vi "Vision Processing.vi"(4 "error in (no error)":errorcluster, 5 "Camera Type":enum16{"206", "1011"}(ring)=enum."1011", 6 "Camera Name":string="Camera") -> ()   [LabVIEW 2013]
uses:
  Robot Global Data.vi
  <vilib>/vision/NI_Vision_Development_Module.lvlib
panel:
  out "Target Info":T1(array[cluster])
  in  "Area Size Limit %":dbl=0.5
  in  "Particle Count Limit":i32=8
  in  "Score Limits":T2={"Rect Coverage"=60.0, "X Edge Strength"=40.0, "Y Edge Strength"=60.0, "Center"=75.0, "Outer"=75.0}
  in  "Processing":enum32{"Color", "Monochrome"}(tab)=enum."Monochrome"
  out "Value":cluster{i32, i32}
  out "Saturation":cluster{i32, i32}
  out "Hue":cluster{i32, i32}
  in  "Luminance":i32=255
  in  "Saturation":i32=255
  in  "Hue":i32(knob)=65 scale=0.0..255.0
  in  "Margins":cluster{"Hue":i32, "Sat":i32, "Val":i32}={"Hue"=33, "Sat"=53, "Val"=9} {"Sat" scale=0.0..80.0; "Val" scale=0.0..80.0; "Hue" scale=0.0..80.0}
  in  "Range":cluster{"Lower value":sgl, "Upper value":sgl}={"Lower value"=150.0, "Upper value"=255.0} {"Lower value" scale=0.0..255.0; "Upper value" scale=0.0..255.0}
  in  "View":bool
  out "Processed Image":T3(plugin-control)
  # "Instructions:\nProcessing the reflective tape that is illuminated by a ring light can be based\non color or light intensity.\nParticles within the image are scored by rectangle coverage, aspect ratio, and\nfor being hollow with a bold edge. A particle is considered a target if all scores\nare above the score limits. Particles can be annotated -- surrounded by\na rectangle and scores drawn to the left .\nTo control the number of particles being scored, use the count limit and the size\nlimit."
  # "To debug, Enable using the View button.\nFor color processing, you can click in the image to select the color for processing."
  # "Enable by clicking the View button.\nGreen scores are above the limit, orange are below. Inner/outer rect\nindicates all passed."
  # "Lower/Upper"
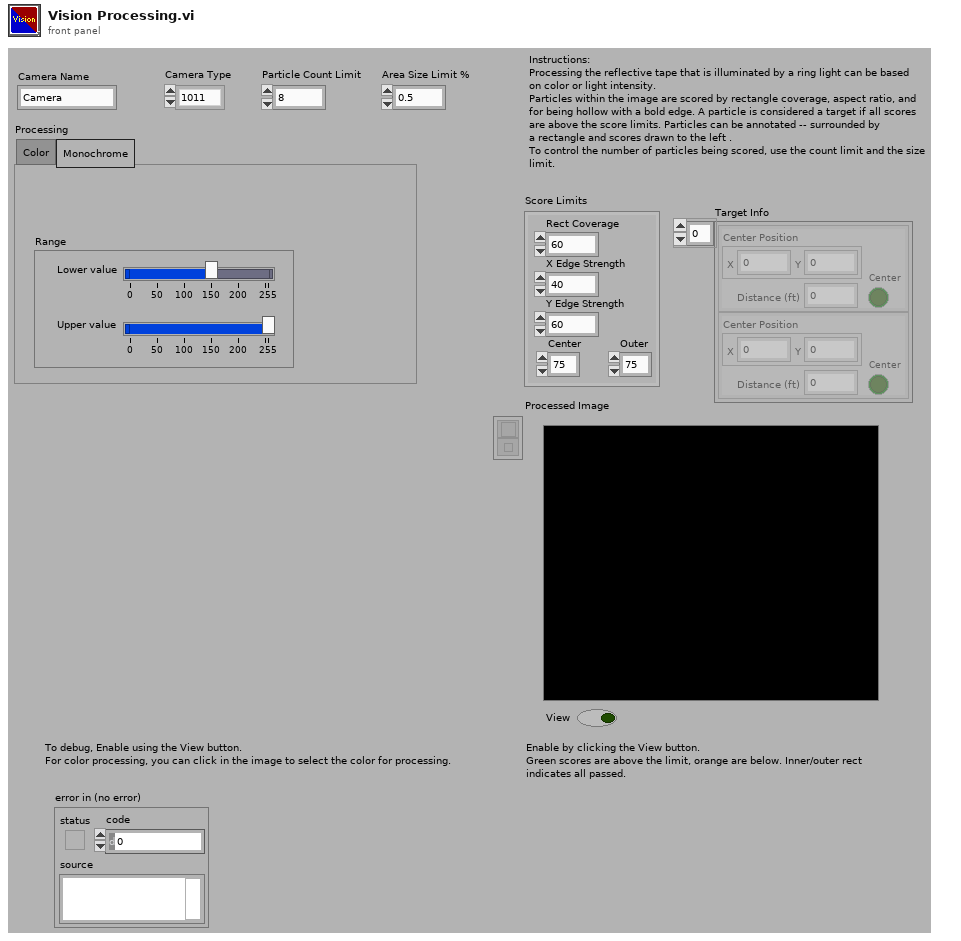
[diagram p1: front panel]
types:
  T1 = cluster{"Center Position":cluster{"X":dbl, "Y":dbl}, "Distance (ft)":dbl, "Center":bool}[]
  T2 = cluster{"Rect Coverage":dbl, "X Edge Strength":dbl, "Y Edge Strength":dbl, "Center":dbl, "Outer":dbl}
  T3 = typedef "IMAQ Image.ctl" = refnum<image>
  T4 = typedef "Image Type" = u32
  T5 = typedef "WPI_CameraDevRef.ctl" = cluster{"Camera Address":string, "CameraStatus":errorcluster, "Acquire Image Notifier":refnum<notifier>}
  T6 = cluster{"Position":cluster{"X":dbl, "Y":dbl}, "Distance (ft)":dbl, "Center":bool}[]
  T7 = typedef "WPI_CameraImageSize.ctl" = enum16{"640x480", "320x240", "160x120"}
  T8 = cluster{cluster{"Left":dbl, "Top":dbl, "Right":dbl, "Bottom":dbl}, "Scores":dbl[], cluster{"Long":dbl, "Short":dbl}}[]
  T9 = cluster{"Target Center (-1 to 1)":cluster{"X":dbl, "Y":dbl}, "Distance (ft)":dbl, "Center Target":bool}
  T10 = cluster{"Target Center (-1 to 1)":cluster{"X":dbl, "Y":dbl}, "Distance (ft)":dbl, "Center Target":bool}[]
  T11 = cluster{"Left":dbl, "Top":dbl, "Right":dbl, "Bottom":dbl}
  T12 = cluster{"Position":cluster{"X":dbl, "Y":dbl}, "Distance (ft)":dbl, "Center":bool}
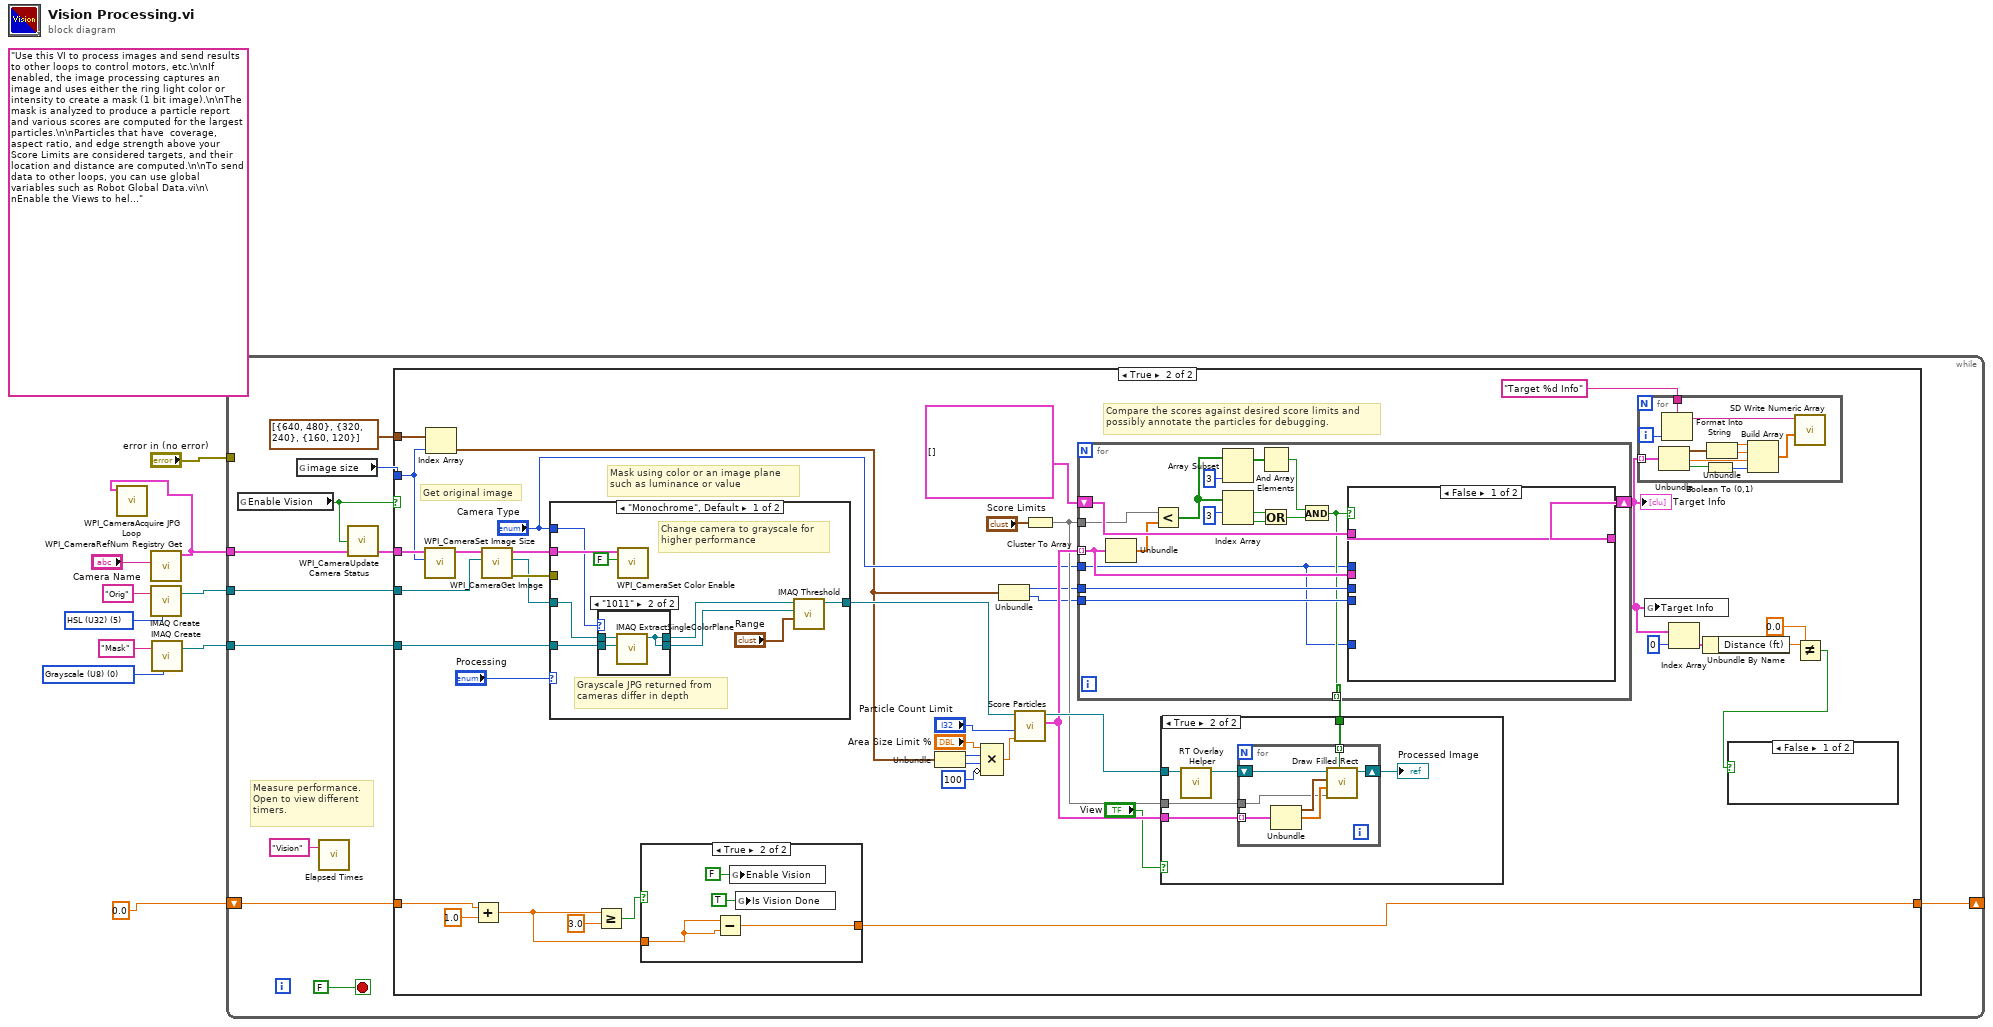
[diagram p0: block diagram]
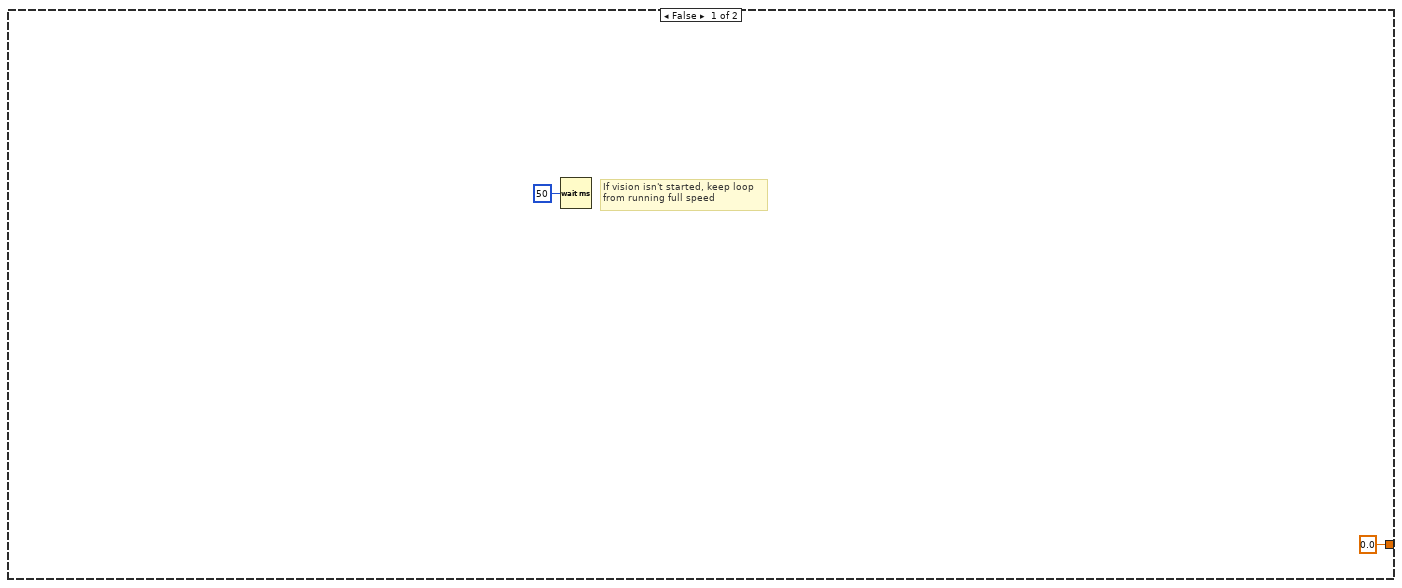
[diagram p2: hidden frame]
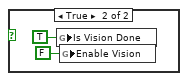
[diagram p3: hidden frame]
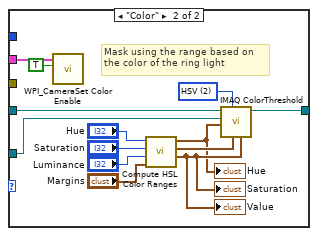
[diagram p6: hidden frame]
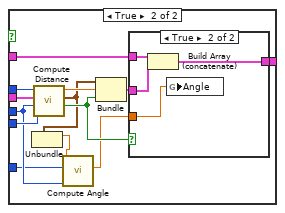
[diagram p8: hidden frame]
diagram:
  w5 = T4 0 items=["Grayscale (U8)", "Grayscale (I16)", "Grayscale (SGL)", "Complex (CSG)", "RGB (U32)", "HSL (U32)", "RGB (U64)", "Grayscale (U16)"] ("Image Type")
  (unwired) "Use this VI to process images and send results to other loops to control motors, etc.\n\nIf enabled, the image processing captures an image and uses either the ring light color or intensity to create a mask (1 bit image).\n\nThe mask is analyzed to produce a particle report and various scores are computed for the largest particles.\n\nParticles that have  coverage, aspect ratio, and edge strength above your Score Limits are considered targets, and their location and distance are computed.\n\nTo send data to other loops, you can use global variables such as Robot Global Data.vi\n\nEnable the Views to help debug color settings. Disable the View to speed up processing."
  w9 = T4 5 items=["Grayscale (U8)", "Grayscale (I16)", "Grayscale (SGL)", "Complex (CSG)", "RGB (U32)", "HSL (U32)", "RGB (U64)", "Grayscale (U16)"] ("Image Type")
  n1 = call <vilib>:"WPI_CameraRefNum Registry Get.vi"("refnum name"="Camera Name") -> ("CameraDevRef"=w1:T5)  [unwired: 9 in, 1 out]
  n2 = call <vilib>:"WPI_CameraAcquire JPG Loop.vi"("CameraDevRef"=w1) -> ()  [unwired: 11 in]
  n3 = call "IMAQ Create"("Image Name"="Orig", "Image Type"=w9) -> ("New Image"=w8:T3)  [unwired: 2 in, 2 out]
  n4 = call "IMAQ Create"("Image Name"="Mask", "Image Type"=w5) -> ("New Image"=w3:T3)  [unwired: 2 in, 2 out]
  n5 = while {
    tunnel: w8 -> [w20]
    tunnel: w1 -> [w19]
    tunnel: "error in (no error)" -> [_]
    tunnel: w3 -> [w14]
    shift-right: [w11] -> _
    shift-left: 0.0 -> [w12]
    stop <- FALSE stop-if-true
    # "Measure performance.\nOpen to view different\ntimers."
    n6 = global read "Robot Global Data.vi" "Enable Vision"() -> (w17:bool)
    n7 = global read "Robot Global Data.vi" "image size"() -> (w15:T7)
    n8 = call "Elapsed Times.vi"("Call Name"="Vision") -> ()  [unwired: 2 in, 1 out]
    n9 = call <vilib>:"WPI_CameraUpdate Camera Status.vi"("CameraDevRef In"=w19, "Enable Vision"=w17) -> ("CameraDevRef Out"=w18:T5)  [unwired: 3 in]
    n10 = case shown="True" w17 {
      tunnel: w20 -> [_ w57]
      tunnel: w18 -> [_ w53]
      tunnel: w15 -> [_ w51]
      tunnel: w14 -> [_ w47]
      tunnel: cluster{i32, i32}[] [{640, 480}, {320, 240}, {160, 120}] -> [_ w50]
      tunnel: w12 -> [_ w34]
      tunnel: [0.0 w30] -> w11
      frame False {
        # "If vision isn't started, keep loop\nfrom running full speed"
        n11 = Wait (ms)(milliseconds to wait=u32 50) -> ()  [unwired: 1 out]
      }
      frame True {
        # "Compare the scores against desired score limits and\npossibly annotate the particles for debugging."
        # "Mask using color or an image plane\nsuch as luminance or value"
        # "Get original image"
        n12 = call <vilib>:"WPI_CameraSet Image Size.vi"("Image Size"=w51, "CameraDevRef"=w53) -> ("CameraDevRef Out"=w54:T5)  [unwired: 8 in, 1 out]
        n13 = Index Array(array=w50, index=w51) -> (element=w36:cluster{i32, i32})
        n14 = Add(x=w34, y=1.0) -> (x+y=w31:dbl)
        n15 = call <vilib>:"WPI_CameraGet Image.vi"("Image"=w57, "CameraDevRef"=w54) -> ("error out"=w55:errorcluster, "Image Out"=w46:T3, "CameraDevRef Out"=w56:T5)  [unwired: 7 in]
        n16 = case shown="\"Monochrome\", Default" "Processing" {
          tunnel: w46 -> [w87 w109]
          tunnel: [w90 w108] -> w52
          tunnel: w56 -> [w88 w101]
          tunnel: w55 -> [_ _]
          tunnel: w47 -> [w86 w99]
          tunnel: "Camera Type" -> [w85 _]
          frame "Monochrome", Default {
            # "Grayscale JPG returned from\ncameras differ in depth"
            # "Change camera to grayscale for\nhigher performance"
            n17 = case shown="\"1011\"" w85 {
              tunnel: w87 -> [w93 w96]
              tunnel: w86 -> [w92 w95]
              tunnel: [w93 w94] -> w84
              tunnel: [w92 w94] -> w83
              frame "206", Default {
              }
              frame "1011" {
                n18 = call "IMAQ ExtractSingleColorPlane"("Image Dst"=w95, "Image Src"=w96) -> ("Image Dst Out"=w94:T3)  [unwired: 8 in, 1 out]
              }
            }
            n19 = call <vilib>:"WPI_CameraSet Color Enable.vi"("Color Enabled"=FALSE, "CameraDevRef"=w88) -> ()  [unwired: 8 in, 2 out]
            n20 = call "IMAQ Threshold"("Range"="Range", "Image Dst"=w83, "Image Src"=w84) -> ("Image Dst Out"=w90:T3)  [unwired: 3 in, 5 out]
          }
          frame "Color" {
            w107 = u16 2 items=["RGB", "HSL", "HSV", "HSI"] ("Color Mode")
            # "Mask using the range based on\nthe color of the ring light"
            n21 = call <vilib>:"WPI_CameraSet Color Enable.vi"("Color Enabled"=TRUE, "CameraDevRef"=w101) -> ()  [unwired: 8 in, 2 out]
            n22 = call "Compute HSL Color Ranges.vi"("Margins"="Margins", "Luminance"="Luminance", "Saturation"="Saturation", "Hue"="Hue") -> ("Lum Range"=w98:cluster{i32, i32}, "Sat Range"=w106:cluster{i32, i32}, "Hue Range"=w97:cluster{i32, i32})  [unwired: 5 in]
            "Hue" <- w97
            "Saturation" <- w98
            "Value" <- w98
            n23 = call "IMAQ ColorThreshold"("Blue or Luma or Val or Inten Range"=w98, "Green or Sat Range"=w106, "Color Mode"=w107, "Red or Hue Range"=w97, "Image Dst"=w99, "Image Src"=w109) -> ("Image Dst Out"=w108:T3)  [unwired: 4 in, 1 out]
          }
        }
        n24 = Greater Or Equal?(x=w31, y=3.0) -> (x >= y?=w32:bool)
        n25 = case shown="True" w32 {
          tunnel: w31 -> [w67 w70]
          tunnel: [w67 w69] -> w30
          frame False {
          }
          frame True {
            n26 = Subtract(x=w70, y=w70) -> (x-y=w69:dbl)
            n27 = global write "Robot Global Data.vi" "Enable Vision"(FALSE ("Enable Vision")) -> ()
            n28 = global write "Robot Global Data.vi" "Is Vision Done"(TRUE ("Is Vision Done")) -> ()
          }
        }
        n29 = Unbundle(w36) -> (w40:i32, w39:i32)
        n30 = Compound Arithmetic op=MULTIPLY("Area Size Limit %", w40, w39, invert 100 ("length")) -> (w37:dbl)
        n31 = Unbundle(w36) -> (w49:i32, w48:i32)
        n32 = call "Score Particles.vi"("Area Size Limit"=w37, "Particle Count Limit"="Particle Count Limit", "Image Refnum in"=w52) -> ("Scored Particle Info"=w61:T8, "Image Refnum out"=w63:T3)  [unwired: 7 in]
        n33 = Cluster To Array(cluster="Score Limits") -> (array=w59:dbl[])
        n34 = for {
          shift-right: [w138] -> w29
          shift-left: T6 [] -> [w139]
          tunnel: w49 -> [w137]
          tunnel: w61 -> [w133] mode=indexing
          tunnel: w59 -> [w135]
          tunnel: "Camera Type" -> [w123]
          tunnel: w48 -> [w134]
          tunnel: [w124] -> w42 mode=indexing
          n35 = Unbundle(w133) -> ("Scores"=w136:dbl[])  [unwired: 2 out]
          n36 = Less?(x=w135, y=w136) -> (x < y?=w125:bool[])
          n37 = Array Subset(array=w125, length=3) -> (w127:bool[])  [unwired: 1 in]
          n38 = Index Array(array=w125, index #1=3 ("length")) -> (element #1=w129:bool, element #2=w130:bool)  [unwired: 1 in]
          n39 = And Array Elements(Boolean array=w127) -> (logical AND=w132:bool)
          n40 = Or(x=w129, y=w130) -> (x .or. y?=w131:bool)
          n41 = And(x=w132, y=w131) -> (x .and. y?=w124:bool)
          n42 = case shown="False" w124 {
            tunnel: w139 -> [w140 w153]
            tunnel: [w140 w152] -> w138
            tunnel: w137 -> [_ w145]
            tunnel: w123 -> [_ w149]
            tunnel: w134 -> [_ w148]
            tunnel: w133 -> [_ w147]
            tunnel: w123 -> [_ w144]
            frame False {
            }
            frame True {
              n43 = call "Compute Distance.vi"("Y Image Resolution"=w148, "X Image Resolution"=w145, "Particle Scores"=w147, "Camera Type"=w149) -> ("Center Target"=w146:bool, "Target Center (-1 to 1)"=w143:cluster{"X":dbl, "Y":dbl}, "Distance (ft)"=w150:dbl)  [unwired: 5 in]
              n44 = Unbundle(w143) -> ("X"=w142:dbl)  [unwired: 1 out]
              n45 = call "Compute Angle.vi"("X Resolution"=w145, "Camera Type"=w144, "X Center (Relative)"=w142) -> ("Angle"=w141:dbl)  [unwired: 8 in]
              n46 = Bundle("Target Center (-1 to 1)"=w143, "Distance (ft)"=w150, "Center Target"=w146) -> (w151:T9)  [unwired: 1 in]
              n47 = case shown="True" w146 {
                tunnel: w153 -> [w154 w158]
                tunnel: [w154 w157] -> w152
                tunnel: w151 -> [_ w156]
                tunnel: w141 -> [_ w155]
                frame False {
                }
                frame True {
                  n48 = Build Array (concatenate)(w158, w156) -> (w157:T10)
                  n49 = global write "Robot Global Data.vi" "Angle"(w155) -> ()
                }
              }
            }
          }
        }
        "Target Info" <- w29
        n50 = case shown="True" "View" {
          tunnel: w63 -> [_ w112]
          tunnel: w61 -> [_ w114]
          tunnel: w59 -> [_ w113]
          tunnel: w42 -> [_ w110]
          frame False {
          }
          frame True {
            n51 = call "RT Overlay Helper.vi"("Refnum in"=w112) -> ("Refnum out"=w115:T3)  [unwired: 10 in]
            n52 = for {
              shift-right: [w121] -> w111
              shift-left: w115 -> [w122]
              tunnel: w114 -> [w118] mode=indexing
              tunnel: w113 -> [w117]
              tunnel: w110 -> [w116] mode=indexing
              n53 = Unbundle(w118) -> (w119:T11, "Scores"=w120:dbl[])  [unwired: 1 out]
              n54 = call "Draw Filled Rect.vi"("Limit Passed"=w116, "Limits"=w117, "Scores"=w120, "Bounding Box"=w119, "image in"=w122) -> ("image out"=w121:T3)  [unwired: 6 in]
            }
            "Processed Image" <- w111
          }
        }
        n55 = for {
          tunnel: w29 -> [w82] mode=indexing
          tunnel: "Target %d Info" ("Name") -> [w81]
          i -> [w78]
          n56 = Unbundle(w82) -> ("Position"=w79:cluster{"X":dbl, "Y":dbl}, "Distance (ft)"=w74:dbl, "Center"=w77:bool)
          n57 = Format Into String(format string=w81, w78) -> (resulting string=w80:string)  [unwired: 2 in, 1 out]
          n58 = Boolean To (0,1)(Boolean=w77) -> (0, 1=w73:i16)
          n59 = Unbundle(w79) -> ("X"=w76:dbl, "Y"=w75:dbl)
          n60 = Build Array(w76, w75, w74, w73) -> (w72:dbl[])
          n61 = call <vilib>:"SD Write Numeric Array.vi"("Numeric Array"=w72, "Name"=w80) -> ()  [unwired: 8 in, 2 out]
        }
        n62 = global write "Robot Global Data.vi" "Target Info"(w29) -> ()
        n63 = Index Array(array=w29, index=0) -> (element=w27:T12)
        n64 = Unbundle By Name(w27) -> ("Distance (ft)"=w26:dbl)
        n65 = Not Equal?(x=w26, y=0.0) -> (x != y?=w24:bool)
        n66 = case shown="False" w24 {
          frame False {
          }
          frame True {
            n67 = global write "Robot Global Data.vi" "Is Vision Done"(TRUE ("Is Vision Done")) -> ()
            n68 = global write "Robot Global Data.vi" "Enable Vision"(FALSE ("Enable Vision")) -> ()
          }
        }
      }
    }
  }
